vi "ACQ Create analog channels.vi"(6 "device in":tag="Dev1", 7 "Config analog chanells new":T1, 8 "error in (no error)":errorcluster, 11 "All Read tasks in":T2) -> (0 "error out":errorcluster, 2 "task out":refnum<k21>, 3 "All Read tasks out":T2, 5 "samples per channel":i32)   [LabVIEW 2014]
doc: "Konfiguruje kanały analogowe dla kanałów:\nAnalog IN - 8 kanałów analogowych\nDigital IN - 4 kanały cyfrowe\nCont IN - 1 kanał przejścia sygnału"
uses:
  Kontrolki/KartaDAQ/ACQ all read tasks.ctl
  Kontrolki/KartaDAQ/ACQ analog channel config new.ctl
  <vilib>/DAQmx/create/channels.llb/DAQmx Create Channel (AI-Voltage-Basic).vi
  <vilib>/DAQmx/configure/timing.llb/DAQmx Timing (Sample Clock).vi
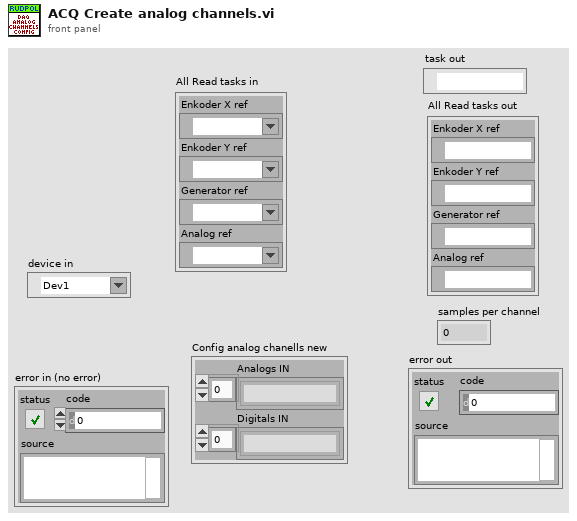
[diagram p1: front panel]
types:
  T1 = typedef "ACQ analog channel config new.ctl" = cluster{"Analogs IN":string[], "Digitals IN":string[]}
  T2 = typedef "ACQ all read tasks.ctl" = cluster{"Enkoder X ref":refnum<k21>, "Enkoder Y ref":refnum<k21>, "Generator ref":refnum<k21>, "Analog ref":refnum<k21>}
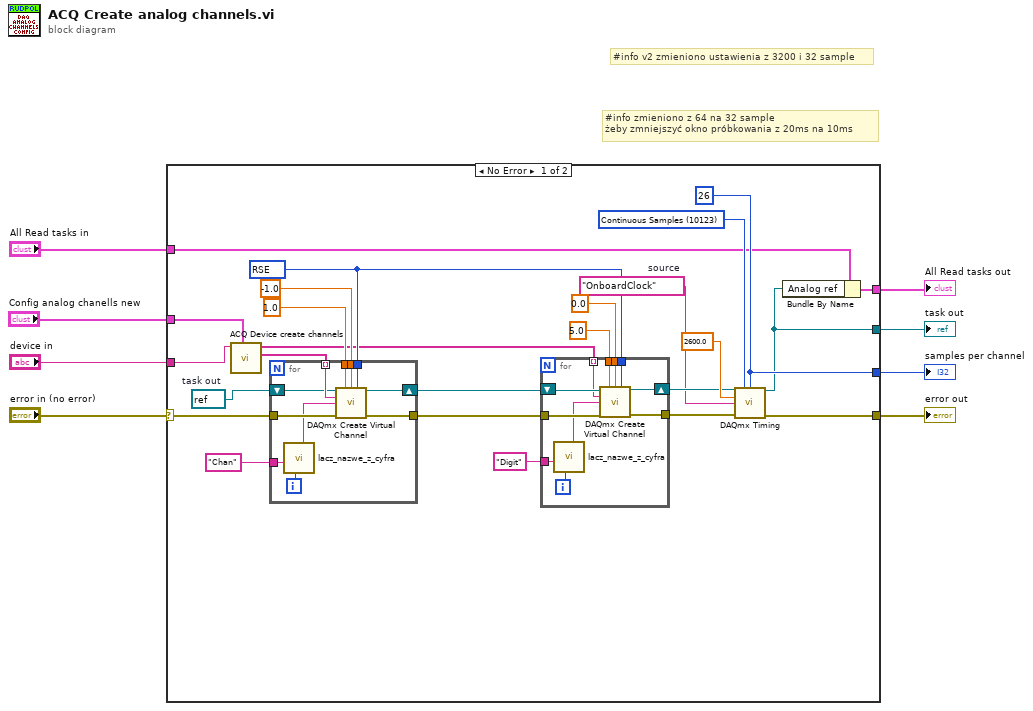
[diagram p0: block diagram]
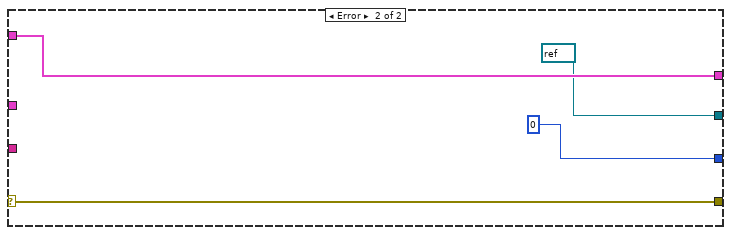
[diagram p2: hidden frame]
diagram:
  # "#info v2 zmieniono ustawienia z 3200 i 32 sample"
  # "#info zmieniono z 64 na 32 sample\nżeby zmniejszyć okno próbkowania z 20ms na 10ms"
  n1 = case shown="No Error" "error in (no error)" {
    selector: "error in (no error)" -> [w25 w59]
    tunnel: [w33 w59] -> w8
    tunnel: [w32 0 ("samples per channel")] -> w7
    tunnel: "device in" -> [w16 _]
    tunnel: "All Read tasks in" -> [w24 w57]
    tunnel: [w23 w57] -> w3
    tunnel: [w22 refnum<k21> refnum ("task out")] -> w2
    tunnel: "Config analog chanells new" -> [w15 _]
    frame No Error {
      w9 = tag "OnboardClock"  # source
      w14 = refnum<k21> refnum  # task out
      w26 = 10123 items=["Finite Samples"=10178, "Continuous Samples"=10123, "Hardware Timed Single Point"=12522] ("sample mode")
      w32 = 26 ("samples per channel")
      w19 = 10083 items=["default"=-1, "RSE"=10083, "NRSE"=10078, "Differential"=10106, "Pseudodifferential"=12529] ("input terminal configuration")
      n2 = call "ACQ Device create channels.vi"("Config analog chanells new"=w15, "device in"=w16) -> ("DAQ analog Array"=w13:tag[], "DAQ digital Array"=w12:tag[])  [unwired: 8 in]
      n3 = for {
        tunnel: 1.0 ("maximum value") -> [w55]
        tunnel: -1.0 ("minimum value") -> [w54]
        tunnel: [w52] -> w28
        tunnel: w25 -> [w51]
        tunnel: w19 -> [w50]
        shift-right: [w53] -> w29
        shift-left: w14 -> [w48]
        tunnel: w13 -> [w49] mode=indexing
        tunnel: "Chan" ("name to assign") -> [w47]
        i -> [w46]
        n4 = call "lacz_nazwe_z_cyfra.vi"("num i"=w46, "name in"=w47) -> ("name out"=w45:string)  [unwired: 9 in]
        n5 = call-poly <vilib>:"DAQmx Create Virtual Channel.vi"("task in"=w48, "maximum value"=w55, "minimum value"=w54, "input terminal configuration"=w50, "physical channels"=w49, "name to assign"=w45, "error in"=w51) -> ("task out"=w53:refnum<k21>, "error out"=w52:errorcluster)  [unwired: 7 in]
      }
      n6 = for {
        tunnel: w28 -> [w43]
        tunnel: 5.0 ("maximum value") -> [w42]
        tunnel: 0.0 ("minimum value") -> [w41]
        tunnel: w19 -> [w40]
        tunnel: [w38] -> w17
        shift-right: [w39] -> w18
        shift-left: w29 -> [w44]
        tunnel: w12 -> [w37] mode=indexing
        tunnel: "Digit" ("name to assign") -> [w35]
        i -> [w36]
        n7 = call "lacz_nazwe_z_cyfra.vi"("num i"=w36, "name in"=w35) -> ("name out"=w34:string)  [unwired: 9 in]
        n8 = call-poly <vilib>:"DAQmx Create Virtual Channel.vi"("task in"=w44, "maximum value"=w42, "minimum value"=w41, "input terminal configuration"=w40, "physical channels"=w37, "name to assign"=w34, "error in"=w43) -> ("task out"=w39:refnum<k21>, "error out"=w38:errorcluster)  [unwired: 7 in]
      }
      n9 = call-poly <vilib>:"DAQmx Timing.vi"("task/channels in"=w18, "sample mode"=w26, "samples per channel"=w32, "rate"=2600.0, "source"=w9, "error in"=w17) -> ("task out"=w22:refnum<k21>, "error out"=w33:errorcluster)  [unwired: 8 in]
      n10 = Bundle By Name(cluster=w24, "Analog ref"=w22) -> (w23:T2)
    }
    frame Error {
    }
  }
  "error out" <- w8
  "samples per channel" <- w7
  "All Read tasks out" <- w3
  "task out" <- w2
